vi "Set Frame Data.vi"(8 "error in":errorcluster, 10 "Data":u8[](array[numeric]), 11 "Frame Ref":T1 format="%.0x") -> (0 "error out":errorcluster, 3 "Frame Ref out":T1 format="%.0x")   [LabVIEW 2020, in "AIM ARINC 664 Scripting.lvlib"]
uses:
  AIM ARINC 664 Scripting.lvlib
  <vilib>/NI VeriStand/Custom Device API/Custom Device API.lvlib
  Constants.vi
  <vilib>/NI VeriStand/Custom Device API/Set Item Property (U32 Array).vi
  <vilib>/NI VeriStand/Custom Device API/Custom Device Item Ref.ctl
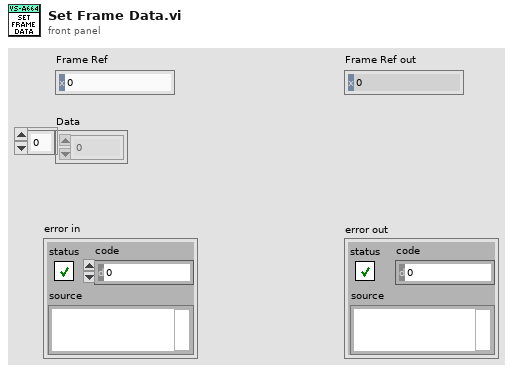
[diagram p1: front panel]
types:
  T1 = typedef "Custom Device API.lvlib/Custom Device Item Ref.ctl" = u64
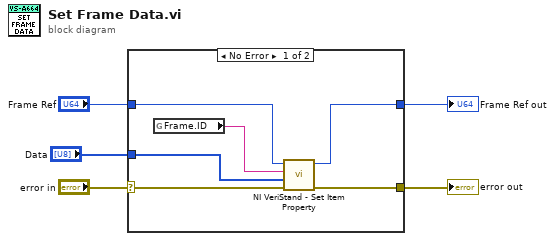
[diagram p0: block diagram]
diagram:
  n1 = case shown="No Error" "error in" {
    selector: "error in" -> [w9 w13]
    tunnel: [w8 w13] -> w4
    tunnel: "Frame Ref" -> [w11 w12]
    tunnel: [w10 w12] -> w2
    tunnel: "Data" -> [w7 _]
    frame No Error {
      n2 = global read "Constants.vi" "Frame.ID"() -> (w6:string)
      n3 = call-poly <vilib>:"NI VeriStand - Set Item Property.vi"("error in (no error)"=w9, "Value"=w7, "Property Name"=w6, "Item Ref in"=w11) -> ("error out"=w8:errorcluster, "Item Ref out"=w10:T1)  [unwired: 5 in, 1 out]
    }
    frame Error {
    }
  }
  "Frame Ref out" <- w2
  "error out" <- w4
